vi "Error Crt Lvl checker.vi"(8 "error in (no error)":errorcluster, 11 "Array of Error Crt in":u8[](array[numeric])) -> (0 "error out":errorcluster, 3 "Array of Error Crt out":u8[](array[numeric]))   [LabVIEW 2026, in "TALOS.lvlib" / "Error Memory.lvlib"]
uses:
  Error Memory.lvlib
  Support VIs/Global Constants.vi
  TALOS.lvlib
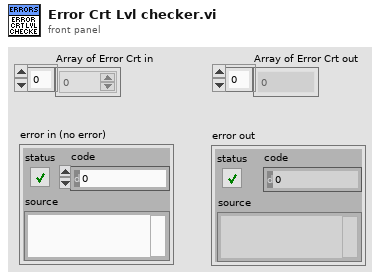
[diagram p1: front panel]
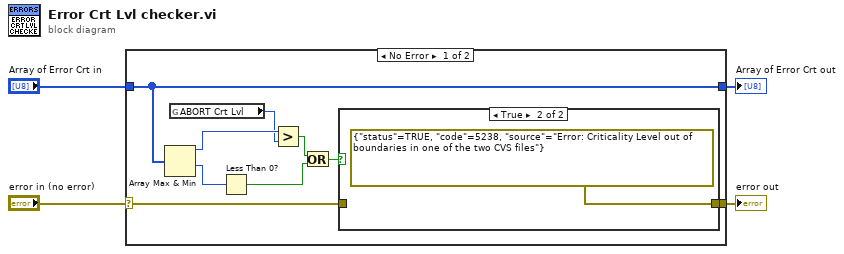
[diagram p0: block diagram]
diagram:
  n1 = case shown="No Error" "error in (no error)" {
    selector: "error in (no error)" -> [w6 w17]
    tunnel: "Array of Error Crt in" -> [w8 w16]
    tunnel: [w5 w17] -> w2
    tunnel: [w8 w16] -> w1
    frame No Error {
      n2 = Array Max & Min(array=w8) -> (max value=w12:u8, min value=w13:u8)  [unwired: 2 out]
      n3 = global read "Global Constants.vi" "ABORT Crt Lvl"() -> (w11:u8)
      n4 = Less Than 0?(x=w13) -> (x < 0?=w9:bool)
      n5 = Greater?(x=w12, y=w11) -> (0:w10:bool)
      n6 = Or(x=w10, y=w9) -> (x .or. y?=w7:bool)
      n7 = case shown="True" w7 {
        tunnel: w6 -> [w14 _]
        tunnel: [w14 errorcluster {"status"=TRUE, "code"=5238, "source"="Error: Criticality Level out of boundaries in one of the two CVS files"} ("error IO")] -> w5
        frame False {
          # "All good!"
        }
        frame True {
        }
      }
    }
    frame Error {
    }
  }
  "Array of Error Crt out" <- w1
  "error out" <- w2
